vi "Write metadata channel.vi"(0 "reference in":refnum<class "TDMS_DataHandler.lvclass">, 2 "channel name":T1, 5 "error in (no error)":errorcluster) -> (14 "reference out":refnum<class "TDMS_DataHandler.lvclass">, 16 "group name out":string, 17 "channel name out":string, 19 "error out":errorcluster)   [LabVIEW 2019, in "TDMS_DataHandler.lvclass"]
doc: "Write the metadata of the given channel of the tdms file"
uses:
  TDMS_DataHandler.lvclass
  Channel names.ctl
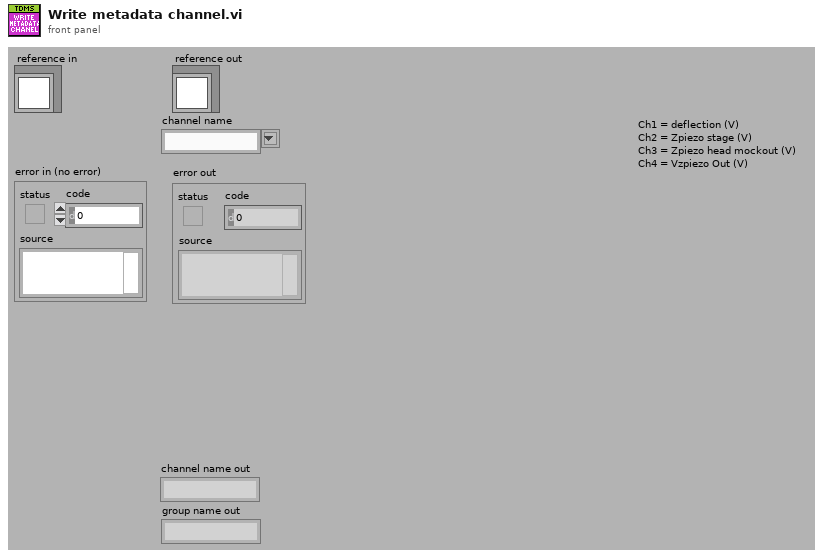
[diagram p1: front panel]
types:
  T1 = typedef "TDMS_DataHandler.lvclass/Channel names.ctl" = string
  T2 = typedef "TDMS_DataHandler.lvclass/ObjectAttributes.ctl" = cluster{"Directory":path, "FilePath":path, "FileRef":refnum<k34>, "ExperimentName":string, "GroupName":string, "ChannelNames":string[], "Datum":waveform(dbl)[], "Group_Metadata":cluster{"property names":string[], "property values":variant[]}, "Channel_Metadata":cluster{"property names":string[], "property values":variant[]}}
  T3 = cluster{"property names":string[], "property values":variant[]}
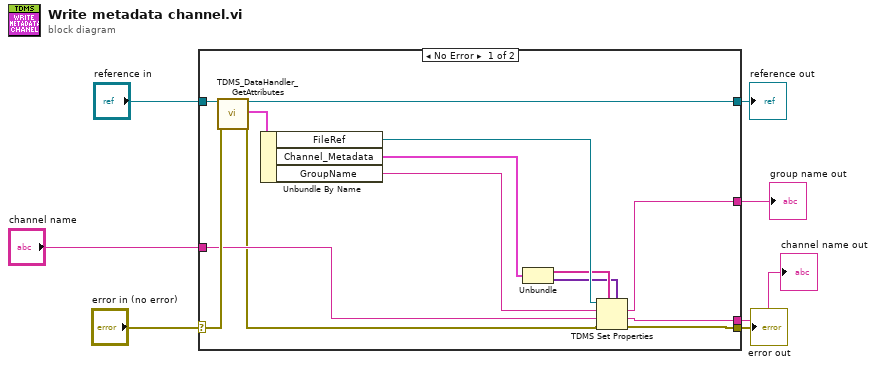
[diagram p0: block diagram]
diagram:
  n1 = case shown="No Error" "error in (no error)" {
    selector: "error in (no error)" -> [w21 w24]
    tunnel: [w11 w24] -> w6
    tunnel: [w20 w23] -> w4
    tunnel: "reference in" -> [w18 w23]
    tunnel: "channel name" -> [w15 w22]
    tunnel: [w14 w22] -> w2
    tunnel: [w13 _] -> w1
    frame No Error {
      n2 = call "TDMS_DataHandler_GetAttributes.vi"("reference in"=w18, "error in (no error)"=w21) -> ("reference out"=w20:refnum<class "TDMS_DataHandler.lvclass">, "attributes"=w19:T2, "error out"=w12:errorcluster)  [unwired: 14 in, 1 out]
      n3 = Unbundle By Name(w19) -> ("FileRef"=w17:refnum<k34>, "Channel_Metadata"=w10:T3, "GroupName"=w16:string)
      n4 = Unbundle(w10) -> ("property names"=w9:string[], "property values"=w8:variant[])
      n5 = TDMS Set Properties(5:w8, 7:w9, 8:w12, 9:w15, 10:w16, 11:w17) -> (0:w11:errorcluster, 1:w14:string, 2:w13:string)  [unwired: 1 out]
    }
    frame Error {
    }
  }
  "error out" <- w6
  "reference out" <- w4
  "channel name out" <- w2
  "group name out" <- w1
